vi "Set Overall Size.vi"(8 "error in":errorcluster, 10 "Overall Size":u32, 11 "Segmented Upload Transfer in":refnum<class "Segmented Upload Transfer.lvclass">) -> (0 "error out":errorcluster, 3 "Segmented Upload Transfer out":refnum<class "Segmented Upload Transfer.lvclass">)   [LabVIEW 2020, in "CANopen.lvlib" / "SDO Manager.lvlib" / "Segmented Upload Transfer.lvclass"]
uses:
  Segmented Upload Transfer.lvclass
  Segmented Upload Transfer.lvclass/Segmented Upload Transfer.ctl
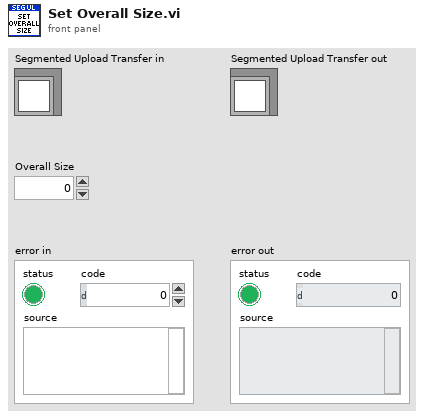
[diagram p1: front panel]
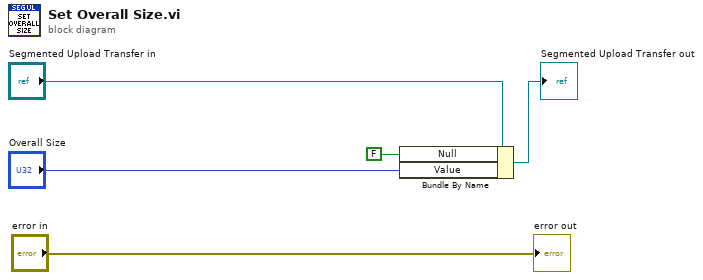
[diagram p0: block diagram]
diagram:
  n1 = Bundle By Name(cluster="Segmented Upload Transfer in", "Null"=FALSE ("Size Indicator.Null"), "Value"="Overall Size") -> (→"Segmented Upload Transfer out":refnum<class "Segmented Upload Transfer.lvclass">)
  "error out" <- "error in"
